vi "test_DevicesDiscover.vi"() -> ()   [LabVIEW 2023]
uses:
  Classes/CCD/CCD.lvclass
  Classes/SCD/SCD.lvclass
  Classes/Mono/Monochromator.lvclass
  <vilib>/addons/_JKI Toolkits/Caraya/classes/Assert/Assert Not Error.vi
  <vilib>/addons/_JKI Toolkits/Caraya/classes/Assert/Assert Equal Value and Type_Variant.vi
  <vilib>/addons/_JKI Toolkits/Caraya/classes/Test/Test.lvclass
  <vilib>/addons/_JKI Toolkits/Caraya/classes/Assert/Assert.lvclass
  Libraries/DeviceManager/DeviceManager.lvlib
panel:
  out "error out":errorcluster
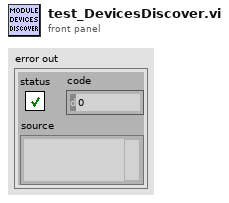
[diagram p1: front panel]
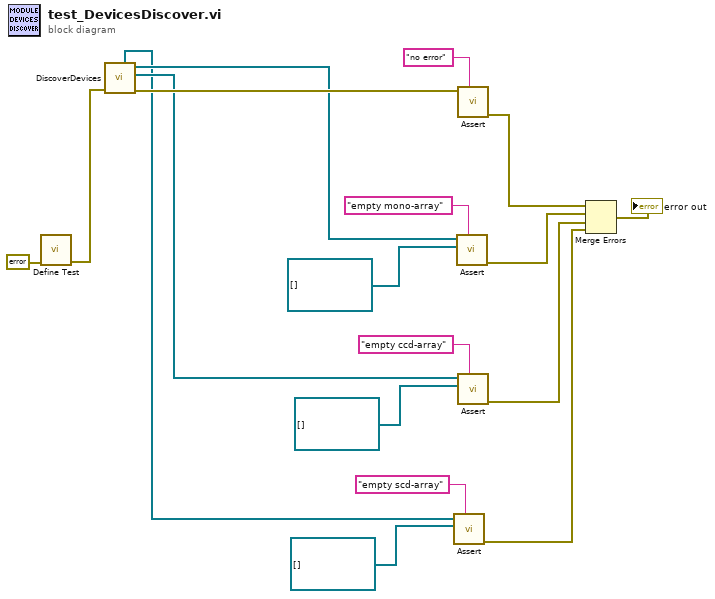
[diagram p0: block diagram]
diagram:
  n1 = call <vilib>:"Define Test.vi"("error in (no error)"=errorcluster {"status"=FALSE, "code"=0, "source"=""}) -> ("error out"=w16:errorcluster)  [unwired: 9 in, 1 out]
  n2 = call "DiscoverDevices.vi"("error in"=w16) -> ("error out"=w13:errorcluster, "CCDs"=w5:refnum<class "CCD.lvclass">[], "Monos"=w4:refnum<class "Monochromator.lvclass">[], "SCDs"=w3:refnum<class "SCD.lvclass">[])  [unwired: 6 in, 1 out]
  n3 = call-poly <vilib>:"Assert.vi"("Label"="empty scd-array" ("Label (VI Title)"), "Y"=refnum<class "SCD.lvclass">[] [] ("CCDs"), "X"=w3) -> ("error out"=w1:errorcluster)  [unwired: 7 in, 1 out]
  n4 = call-poly <vilib>:"Assert.vi"("Label"="empty mono-array" ("Label (VI Title)"), "Y"=refnum<class "Monochromator.lvclass">[] [] ("Array"), "X"=w4) -> ("error out"=w11:errorcluster)  [unwired: 7 in, 1 out]
  n5 = call-poly <vilib>:"Assert.vi"("Label"="no error" ("Label (VI Title)"), "Not Error?"=w13) -> ("error out"=w14:errorcluster)  [unwired: 8 in, 1 out]
  n6 = call-poly <vilib>:"Assert.vi"("Label"="empty ccd-array" ("Label (VI Title)"), "Y"=refnum<class "CCD.lvclass">[] [] ("CCDs"), "X"=w5) -> ("error out"=w2:errorcluster)  [unwired: 7 in, 1 out]
  n7 = Merge Errors(w14, w11, w2, w1) -> (→"error out":errorcluster)
